vi "Read Rank.vi"(8 "error in (no error)":errorcluster, 11 "Vector 26GHz Path Group in":refnum<class "Vector 26GHz Path Group.lvclass">) -> (0 "error out":errorcluster, 2 "Rank":dbl, 3 "Vector 26GHz Path Group out":refnum<class "Vector 26GHz Path Group.lvclass">)   [LabVIEW 2023, in "RFFixtureCharact.RMM.lvlib" / "Vector 26GHz Path Group.lvclass"]
uses:
  Vector 26GHz Path Group.lvclass
  Vector 26GHz Path Group.lvclass/Vector 26GHz Path Group.ctl
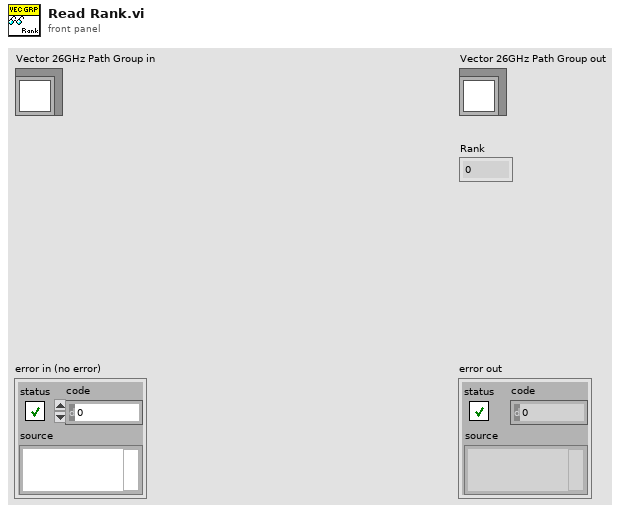
[diagram p1: front panel]
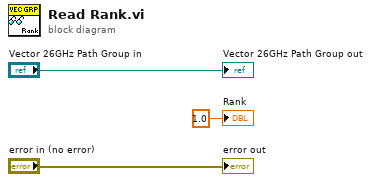
[diagram p0: block diagram]
diagram:
  "error out" <- "error in (no error)"
  "Vector 26GHz Path Group out" <- "Vector 26GHz Path Group in"
  "Rank" <- 1.0 ("Rank")
